vi "Set Reset Flip Flop.vi"(7 "Reset":bool, 11 "Set":bool) -> (3 "Out":bool)   [LabVIEW 2014]
panel:
  # "Copyright 2014 Vidrio Technologies\nScanImage 5 software is licensed under the Apache License, Version 2.0 (the \"License\"); you may not use any files contained\nwithin the ScanImage 5 release except in compliance with the License. You may obtain a copy of the License at\n http://www.apache.org/licenses/LICENSE-2.0\nUnless required by applicable law or agreed to in writing, software distributed under the License is distributed on an\n\"AS IS\" BASIS, WITHOUT WARRANTIES OR CONDITIONS OF ANY KIND, either express or implied. See the License for the\n specific language governing permissions and limitations under the License."
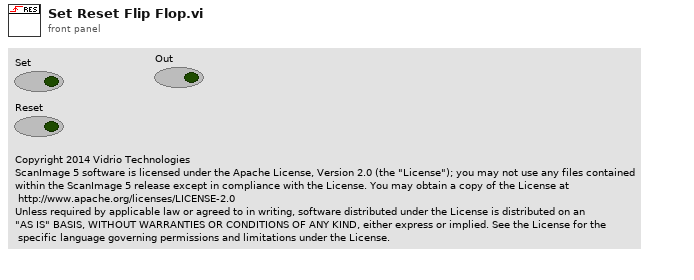
[diagram p1: front panel]
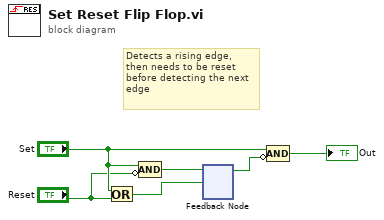
[diagram p0: block diagram]
diagram:
  # "Detects a rising edge,\nthen needs to be reset\nbefore detecting the next\nedge"
  n1 = Or(x="Set", y="Reset") -> (x .or. y?=w5:bool)
  n2 = Compound Arithmetic op=AND("Set", invert "Reset") -> (w3:bool)
  n3 = feedback #1() -> (w6:bool)  [unwired: 1 in]
  n4 = feedback-in #1(w3, w5) -> ()
  n5 = Compound Arithmetic op=AND("Set", invert w6) -> (→"Out":bool)
